vi "Copy Value.vi"(8 "error in (no error)":errorcluster, 10 "From":refnum<class "Type.lvclass">, 11 "Entity in":refnum<class "Entity C.lvclass">) -> (0 "error out":errorcluster, 3 "Entity out":refnum<class "Entity C.lvclass">)   [LabVIEW 2020, in "Conditum.lvlib" / "Columns.lvlib" / "Entity C.lvclass"]
uses:
  Entity C.lvclass
  Type/Type.lvclass
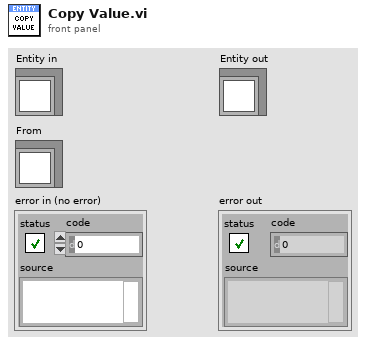
[diagram p1: front panel]
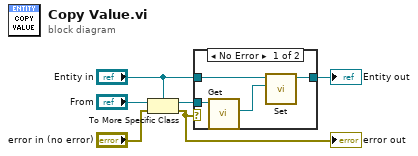
[diagram p0: block diagram]
diagram:
  n1 = To More Specific Class(target class="Entity in", reference="From", error in="error in (no error)") -> (specific class reference=w6:refnum<class "Entity C.lvclass">, error out=w2:errorcluster)
  "error out" <- w2
  n2 = case shown="No Error" w2 {
    tunnel: w6 -> [w10 _]
    tunnel: "Entity in" -> [w8 w11]
    tunnel: [w7 w11] -> w1
    frame No Error {
      n3 = call "Get.vi"("Entity in"=w10) -> ("Value"=w9:refnum<class "Entity.lvclass">)  [unwired: 10 in]
      n4 = call "Set.vi"("Value"=w9, "Entity in"=w8) -> ("Entity out"=w7:refnum<class "Entity C.lvclass">)  [unwired: 9 in]
    }
    frame Error {
    }
  }
  "Entity out" <- w1
